vi "_Measure Transfer Function.vi"() -> ()   [LabVIEW 2014]
panel:
  out "VISA Refnum out":refnum<visa-resource-name>
  out "error out":errorcluster
  in  "#Samples to read":i32
  out "Output":u16(graph)
  in  "VISA Refnum in":refnum<visa-resource-name>
  in  "error in":errorcluster
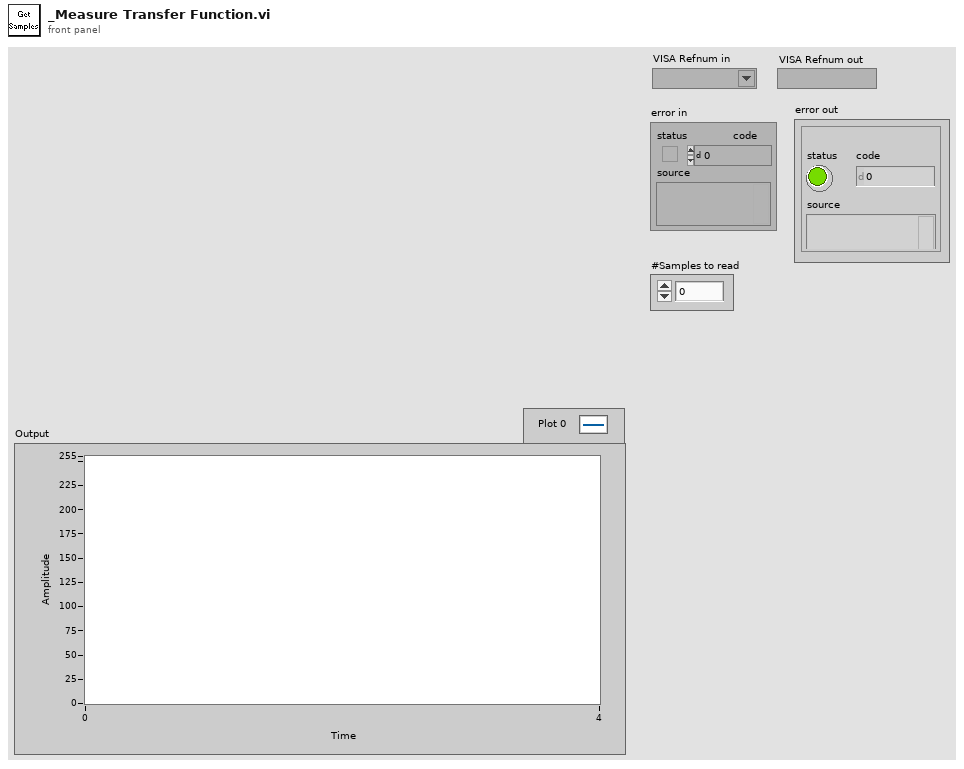
[diagram p1: front panel]
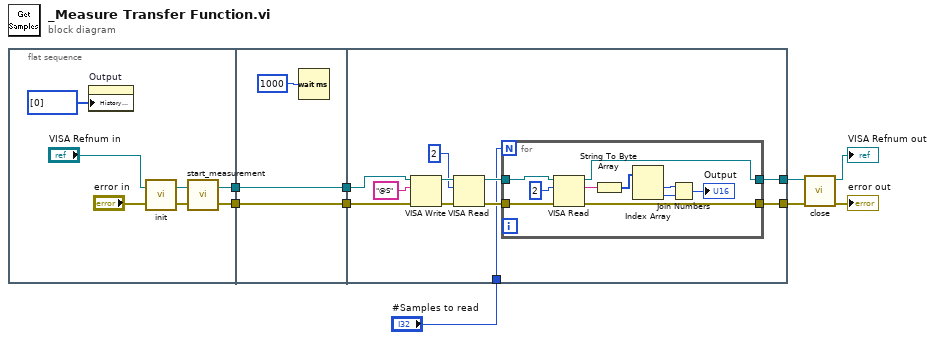
[diagram p0: block diagram]
diagram:
  n1 = flat-sequence {
    tunnel: [w16] -> w8
    tunnel: [w15] -> w6
    tunnel: w8 -> [w19]
    tunnel: [w19] -> w7
    tunnel: w6 -> [w18]
    tunnel: [w18] -> w5
    tunnel: w5 -> [w22]
    tunnel: w7 -> [w23]
    tunnel: "#Samples to read" -> [w24]
    tunnel: [w21] -> w2
    tunnel: [w20] -> w1
    frame #0 {
      n2 = property on="Output" class="WFChart (strict)"("History Data"=u8[] [0]) -> ()  [unwired: 2 in, 2 out]
      n3 = call "init.vi"("error in (no error)"="error in", "VISA Refnum in"="VISA Refnum in") -> ("error out"=w11:errorcluster, "VISA Refnum out"=w10:refnum<visa-resource-name>)
      n4 = call "start_measurement.vi"("error in (no error)"=w11, "VISA Refnum in"=w10) -> ("error out"=w15:errorcluster, "VISA Refnum out"=w16:refnum<visa-resource-name>)
    }
    frame #1 {
      n5 = Wait (ms)(milliseconds to wait=u32 1000) -> ()  [unwired: 1 out]
    }
    frame #2 {
      n6 = VISA Write(VISA resource name=w23, write buffer="@S", error in (no error)=w22) -> (VISA resource name out=w27:refnum<visa-resource-name>, error out=w26:errorcluster)  [unwired: 1 out]
      n7 = VISA Read(VISA resource name=w27, byte count=u32 2, error in (no error)=w26) -> (VISA resource name out=w29:refnum<visa-resource-name>, error out=w30:errorcluster)  [unwired: 2 out]
      n8 = for {
        N: w24 -> [_]
        tunnel: w29 -> [w39]
        tunnel: w30 -> [w40]
        tunnel: [w32] -> w21
        tunnel: [w31] -> w20
        n9 = VISA Read(VISA resource name=w39, byte count=u32 2, error in (no error)=w40) -> (VISA resource name out=w32:refnum<visa-resource-name>, read buffer=w33:string, error out=w31:errorcluster)  [unwired: 1 out]
        n10 = String To Byte Array(string=w33) -> (unsigned byte array=w37:u8[])
        n11 = Index Array(array=w37) -> (element #1=w36:u8, element #2=w35:u8)  [unwired: 2 in]
        n12 = Join Numbers(hi=w36, lo=w35) -> ((hi.lo)=→"Output":u16)
      }
    }
  }
  n13 = call "close.vi"("error in (no error)"=w1, "VISA resource name"=w2) -> ("error out"=→"error out":errorcluster, "VISA resource name out"=→"VISA Refnum out":refnum<visa-resource-name>)  [unwired: 4 in]
